vi "LabGUI Launcher.vi"   [LabVIEW 2019, in "LabGUI.lvlib"]
uses:
  LabGUI.lvlib
  LabGUI/LabGUI.lvclass
  C:/Program Files (x86)/National Instruments/LabVIEW 2019/vi.lib/MGI/Panel Manager/Panel Actor/Panel Actor/Panel Actor.lvclass
  <vilib>/MGI/Panel Manager/Panel/Window Position/Reference Position/Alignment.ctl
  <vilib>/MGI/Panel Manager/Panel/Window Position/Reference Position/Horizontal Alignment.ctl
  <vilib>/MGI/Panel Manager/Panel/Window Position/Reference Position/Vertical Alignment.ctl
  <vilib>/MGI/Panel Manager/Panel/Window Position/Reference Position/Offset/Absolute Offset/Absolute Offset.lvclass
  C:/Program Files (x86)/National Instruments/LabVIEW 2019/vi.lib/MGI/Panel Manager/Panel/Window Position/Reference Position/Offset/Offset.lvclass
  <vilib>/MGI/Panel Manager/Panel/Window Position/Reference Position/Ref Display/Ref Display.lvclass
  C:/Program Files (x86)/National Instruments/LabVIEW 2019/vi.lib/MGI/Panel Manager/Panel/Window Position/Window Position.lvclass
  <vilib>/MGI/Panel Manager/Panel Actor/Panel Actor/Launch Root Panel Window.vi
  <vilib>/MGI/Panel Manager/Panel/Window Position/Reference Position/Ref Display/Ref Display.vi
  <vilib>/MGI/Panel Manager/Panel/Window Position/Reference Position/Offset/Absolute Offset/No Offset.vi
  <vilib>/MGI/Panel Manager/Panel Actor/Panel Actor/Panel Actor.lvclass
  <vilib>/MGI/Panel Manager/Panel/Panel.lvlib
  <vilib>/MGI/Panel Manager/Panel/Window Position/Reference Position/Reference Position.lvclass
  C:/Program Files (x86)/National Instruments/LabVIEW 2019/vi.lib/MGI/Panel Manager/Panel/Window Position/Reference Position/Reference Position.lvclass
  C:/Program Files (x86)/National Instruments/LabVIEW 2019/vi.lib/MGI/Monitored Actor/Monitored Actor/Monitored Actor/Monitored Actor.lvclass
  C:/Program Files (x86)/National Instruments/LabVIEW 2019/vi.lib/ActorFramework/Actor/Actor.lvclass
panel:
  # "LabGUI"
types:
  T1 = enum32{"Invalid", "Standard", "Closed", "Hidden", "Minimized", "Maximized"}
  T2 = typedef "Panel.lvlib/Reference Position.lvclass/Alignment.ctl" = cluster{"Horizontal":T3, "Vertical":T4}
  T3 = typedef "Panel.lvlib/Reference Position.lvclass/Horizontal Alignment.ctl" = enum16{"Left", "Center", "Right"}
  T4 = typedef "Panel.lvlib/Reference Position.lvclass/Vertical Alignment.ctl" = enum16{"Top", "Center", "Bottom"}
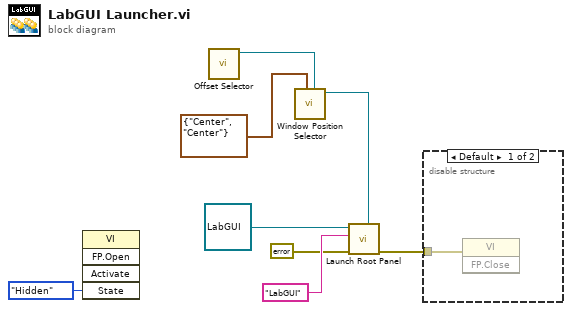
[diagram p0: block diagram]
diagram:
  n1 = invoke class="VI" method="FP.Open"("State"=T1."Hidden") -> ()  [unwired: 4 in, 5 out]
  n2 = call-poly <vilib>:"Offset Selector.vi"() -> ("Absolute Offset Out"=w2:refnum<class "Absolute Offset.lvclass">)  [unwired: 10 in, 1 out]
  n3 = call-poly <vilib>:"Window Position Selector.vi"("Offset"=w2, "Alignment"=T2 {"Horizontal"=enum."Center", "Vertical"=enum."Center"}) -> ("Ref Display out"=w6:refnum<class "Ref Display.lvclass">)  [unwired: 8 in, 1 out]
  n4 = call-poly <vilib>:"Launch Root Panel.vi"("Window Position (Maximize First Call)"=w6, "Error In"=errorcluster {"status"=FALSE, "code"=0, "source"=""} ("error in (no error)"), "Title"="LabGUI", "Panel Actor in"=refnum<class "LabGUI.lvclass"> refnum ("LabGUI.lvlib:LabGUI.lvclass")) -> ("Error Out"=w7:errorcluster)  [unwired: 6 in, 1 out]
  n5 = disable-structure shown="Default" {
    disable-tunnel: w7 -> [w9 _]
    frame condition #0 {
      n6 = invoke class="VI" method="FP.Close"(error in=w9) -> ()  [unwired: 2 in, 3 out]
    }
    frame condition #1 (active) {
    }
  }
